vi "thermalCamera.vi"() -> ()   [LabVIEW 2025]
panel:
  out "Image":T1(plugin-control)
  out "IP address":string
  in  "Stop Button":bool
  out "Output":string
  in  "Flag":bool
  in  "Stop recording":bool
  in  "Stop Preview":bool
  in  "Focus":dbl(slide) scale=0.0..100.0
  in  "Record":bool
  in  "Connect Server":bool
  out "?":string
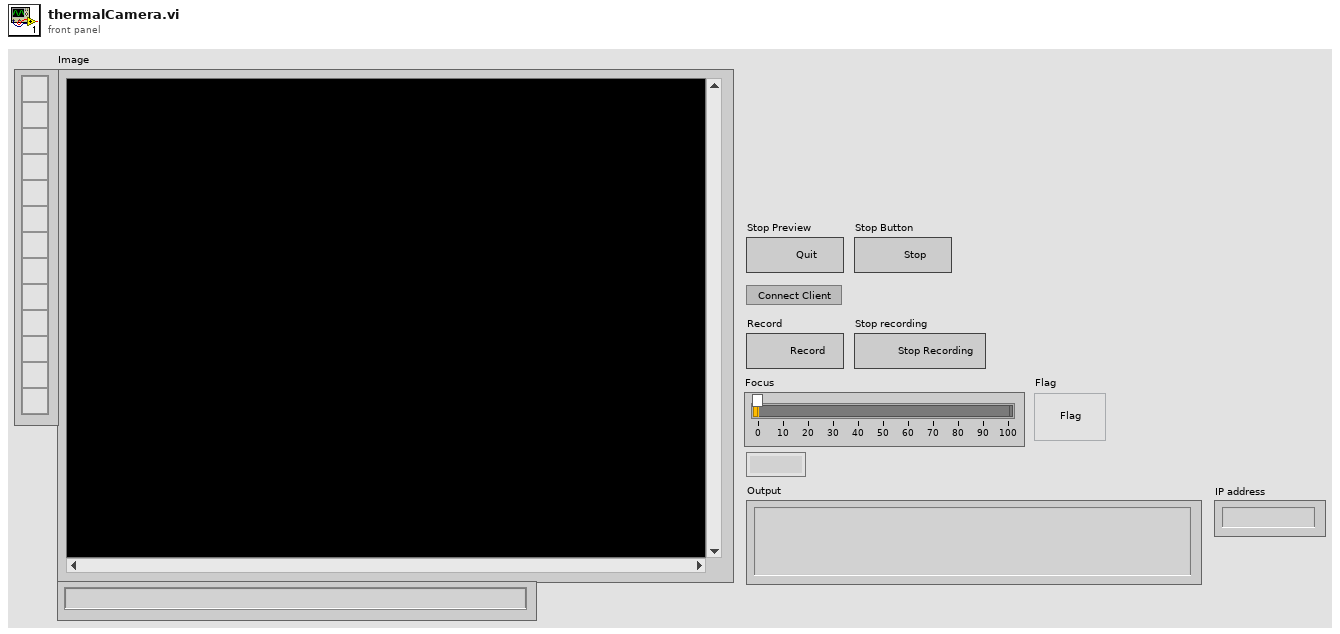
[diagram p1: front panel]
types:
  T1 = typedef "IMAQ Image.ctl" = refnum<image>
  T2 = enum16{"open", "replace", "create", "open or create", "replace or create", "replace or create with confirmation"}
  T3 = enum16{"big-endian, network order", "native, host order", "little-endian"}
  T4 = enum16{"Standard", "Buffered", "CRLF", "Immediate"}
  T5 = typedef "Image Type" = u32
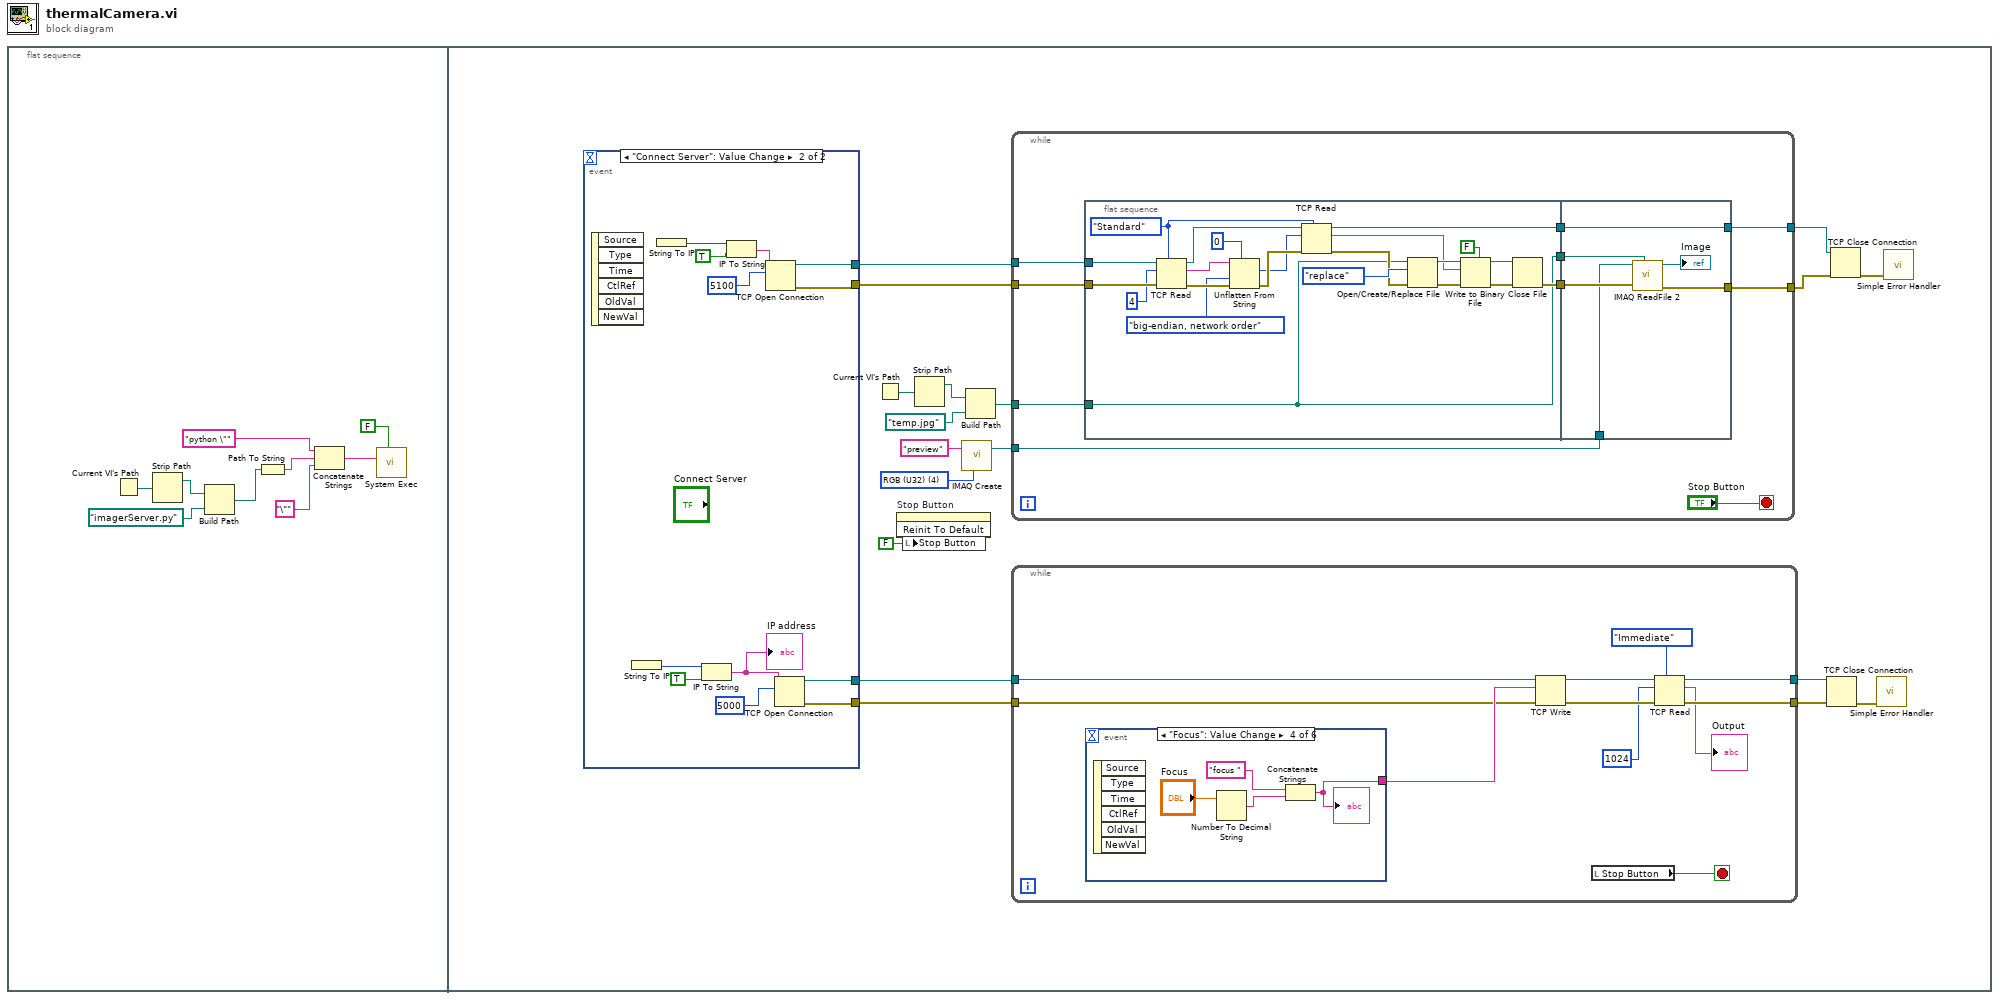
[diagram p0: block diagram]
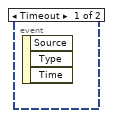
[diagram p2: hidden frame]
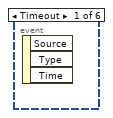
[diagram p3: hidden frame]
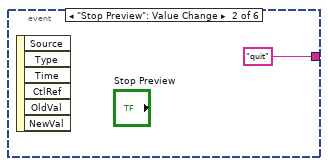
[diagram p4: hidden frame]
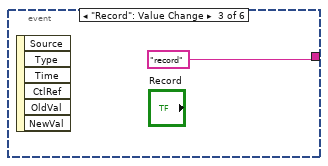
[diagram p5: hidden frame]
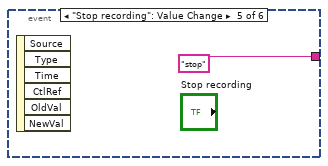
[diagram p6: hidden frame]
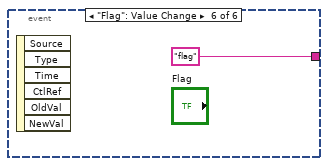
[diagram p7: hidden frame]
diagram:
  n1 = flat-sequence {
    frame #0 {
      n2 = Current VI's Path() -> (path=w4:path)
      n3 = Strip Path(path=w4) -> (stripped path=w5:path)  [unwired: 1 out]
      n4 = Build Path(base path=w5, name or relative path=path "imagerServer.py") -> (appended path=w2:path)
      n5 = Path To String(path=w2) -> (string=w8:string)
      n6 = Concatenate Strings("python \"" ("string"), w8, "\"" ("string")) -> (w7:string)
      n7 = call <vilib>:"System Exec.vi"("wait until completion? (T)"=FALSE, "command line"=w7) -> ()  [unwired: 6 in, 4 out]
    }
    frame #1 {
      w13 = T5 4 items=["Grayscale (U8)", "Grayscale (I16)", "Grayscale (SGL)", "Complex (CSG)", "RGB (U32)", "HSL (U32)", "RGB (U64)", "Grayscale (U16)"] ("Image Type")
      n8 = event shown="[1] \"Connect Server\": Value Change" {
        selector: _ -> [_ _]
        dyn-events: _ -> [_ _]
        timeout: _ -> [_ _]
        tunnel: [_ w38] -> w24
        tunnel: [_ w37] -> w23
        tunnel: [_ w29] -> w12
        tunnel: [_ w28] -> w11
        event Timeout {
          n9 = event-data() -> ()  [unwired: 1 in, 3 out]
        }
        event "Connect Server": Value Change {
          n10 = event-data() -> ()  [unwired: 1 in, 6 out]
          n11 = String To IP() -> (0:w32:u32)  [unwired: 1 in]
          n12 = String To IP() -> (0:w36:u32)  [unwired: 1 in]
          n13 = IP To String(1:TRUE ("dot notation? (F)"), 2:w32) -> (0:w33:string)
          "IP address" <- w33
          n14 = IP To String(1:TRUE ("dot notation? (F)"), 2:w36) -> (0:w34:string)
          n15 = TCP Open Connection(address=w34, remote port or service name=u16 5100) -> (connection ID=w37:refnum<k5>, error out=w38:errorcluster)  [unwired: 3 in]
          n16 = TCP Open Connection(address=w33, remote port or service name=u16 5000) -> (connection ID=w28:refnum<k5>, error out=w29:errorcluster)  [unwired: 3 in]
        }
      }
      n17 = Current VI's Path() -> (path=w26:path)
      n18 = invoke on="Stop Button" class="Bool (strict)" method="Reinit To Default"() -> ()  [unwired: 3 in, 3 out]
      n19 = local write "Stop Button"(FALSE ("Stop Button")) -> ()
      n20 = Strip Path(path=w26) -> (stripped path=w27:path)  [unwired: 1 out]
      n21 = call "IMAQ Create"("Image Name"="preview", "Image Type"=w13) -> ("New Image"=w20:T1)  [unwired: 3 in, 1 out]
      n22 = Build Path(base path=w27, name or relative path=path "temp.jpg") -> (appended path=w25:path)
      n23 = while {
        tunnel: w20 -> [w42]
        tunnel: w24 -> [w48]
        tunnel: w23 -> [w49]
        tunnel: [w43] -> w21
        tunnel: [w47] -> w22
        tunnel: w25 -> [w45]
        stop <- "Stop Button" stop-if-true
        n24 = flat-sequence {
          tunnel: w49 -> [w71]
          tunnel: w48 -> [w70]
          tunnel: w45 -> [w51]
          tunnel: [w53] -> w46
          tunnel: [w52] -> w44
          tunnel: [w51] -> w41
          tunnel: [w77] -> w47
          tunnel: w46 -> [w77]
          tunnel: w44 -> [w76]
          tunnel: [w75] -> w43
          tunnel: w42 -> [w74]
          tunnel: w41 -> [w73]
          frame #0 {
            w62 = T4."Standard" ("mode (standard)")
            n25 = TCP Read(connection ID=w71, bytes to read=4, error in (no error)=w70, 7:w62) -> (connection ID out=w65:refnum<k5>, data out=w50:string, error out=w68:errorcluster)  [unwired: 1 in]
            n26 = Unflatten From String(type=0, binary string=w50, byte order (0:big-endian, network order)=T3."big-endian, network order", error in (no error)=w68) -> (value=w63:i32, error out=w64:errorcluster)  [unwired: 1 in, 1 out]
            n27 = TCP Read(connection ID=w65, bytes to read=w63, error in (no error)=w64, 7:w62) -> (connection ID out=w53:refnum<k5>, data out=w58:string, error out=w60:errorcluster)  [unwired: 1 in]
            n28 = Open/Create/Replace File(file path (use dialog)=w51, error in=w60, operation (0:open)=T2."replace") -> (refnum out=w59:refnum<file>, error out=w56:errorcluster)  [unwired: 3 in, 1 out]
            n29 = Write to Binary File(file (use dialog)=w59, data=w58, error in=w56, 5:FALSE ("prepend array or string size? (T)")) -> (refnum out=w54:refnum<file>, error out=w55:errorcluster)  [unwired: 2 in, 1 out]
            n30 = Close File(refnum=w54, error in=w55) -> (error out=w52:errorcluster)  [unwired: 1 out]
          }
          frame #1 {
            n31 = call "IMAQ ReadFile 2"("File Path"=w73, "error in (no error)"=w76, "Image"=w74) -> ("error out"=w75:errorcluster, "Image Out"=→"Image":T1)  [unwired: 4 in, 3 out]
          }
        }
      }
      n32 = while {
        tunnel: [w87] -> w16
        tunnel: [w85] -> w17
        tunnel: w12 -> [w83]
        tunnel: w11 -> [w82]
        stop <- w78 stop-if-true
        n33 = event shown="[3] \"Focus\": Value Change" {
          selector: _ -> [_ _ _ _ _ _]
          dyn-events: _ -> [_ _ _ _ _ _]
          timeout: _ -> [_ _ _ _ _ _]
          tunnel: [_ "quit" "record" w92 "stop" "flag"] -> w84
          event Timeout {
            n34 = event-data() -> ()  [unwired: 1 in, 3 out]
          }
          event "Stop Preview": Value Change {
            n35 = event-data() -> ()  [unwired: 1 in, 6 out]
          }
          event "Record": Value Change {
            n36 = event-data() -> ()  [unwired: 1 in, 6 out]
          }
          event "Focus": Value Change {
            n37 = event-data() -> ()  [unwired: 1 in, 6 out]
            n38 = Number To Decimal String(number="Focus") -> (decimal integer string=w94:string)  [unwired: 1 in]
            n39 = Concatenate Strings("focus ", w94) -> (w92:string)
            "?" <- w92
          }
          event "Stop recording": Value Change {
            n40 = event-data() -> ()  [unwired: 1 in, 6 out]
          }
          event "Flag": Value Change {
            n41 = event-data() -> ()  [unwired: 1 in, 6 out]
          }
        }
        n42 = TCP Write(connection ID=w82, data in=w84, error in (no error)=w83) -> (connection ID out=w86:refnum<k5>, error out=w88:errorcluster)  [unwired: 1 in, 1 out]
        n43 = local read "Stop Button"() -> (w78:bool)
        n44 = TCP Read(connection ID=w86, bytes to read=1024, error in (no error)=w88, 7:T4."Immediate" ("mode (standard)")) -> (connection ID out=w85:refnum<k5>, data out=→"Output":string, error out=w87:errorcluster)  [unwired: 1 in]
      }
      n45 = TCP Close Connection(connection ID=w17, error in (no error)=w16) -> (error out=w18:errorcluster)  [unwired: 1 in, 1 out]
      n46 = TCP Close Connection(connection ID=w22, error in (no error)=w21) -> (error out=w19:errorcluster)  [unwired: 1 in, 1 out]
      n47 = call <vilib>:"Simple Error Handler.vi"("error in (no error)"=w18) -> ()  [unwired: 4 in, 5 out]
      n48 = call <vilib>:"Simple Error Handler.vi"("error in (no error)"=w19) -> ()  [unwired: 4 in, 5 out]
    }
  }
